vi "Eurotherm_PID_Simplified.vi"() -> ()   [LabVIEW 2013]
uses:
  <vilib>/Utility/file.llb/Write To Spreadsheet File (string).vi
  <vilib>/Utility/file.llb/Write To Spreadsheet File (DBL).vi
panel:
  in  "Ramp-Down Rate(°C/ min)":dbl
  in  "Target Setpoint (°C)":sgl format="%#.1f"
  in  "RAMP":bool
  in  "Dwell Time (min)":dbl
  in  "Ramp-Up Rate (°C/ min)":dbl
  in  "SET":bool
  in  "DELAY":u32=300 caption="ms"
  in  "Save Button":bool
  in  "File Path":path
  in  "Sample":string
  in  "User":string
  out "Time":dbl caption="(s)"
  in  "Setpoint Value":sgl min=0 max=1300 format="%.3f"
  in  "SET PID":bool
  in  "P":sgl=1.0
  in  "I":u32=10000
  in  "D":u32=1000
  in  "Controller Mode":u8(ring) items=["Auto", "Manual"]
  in  "stop":bool
  out "Temperature":cluster{dbl[], sgl[]}(graph)
  out "Temperature":sgl caption="°C" format="%.3g"
  in  "Unit":u8=1
  in  "VISA resource name":refnum<visa-resource-name>="COM4"
  # "Configuration - Requires Restart"
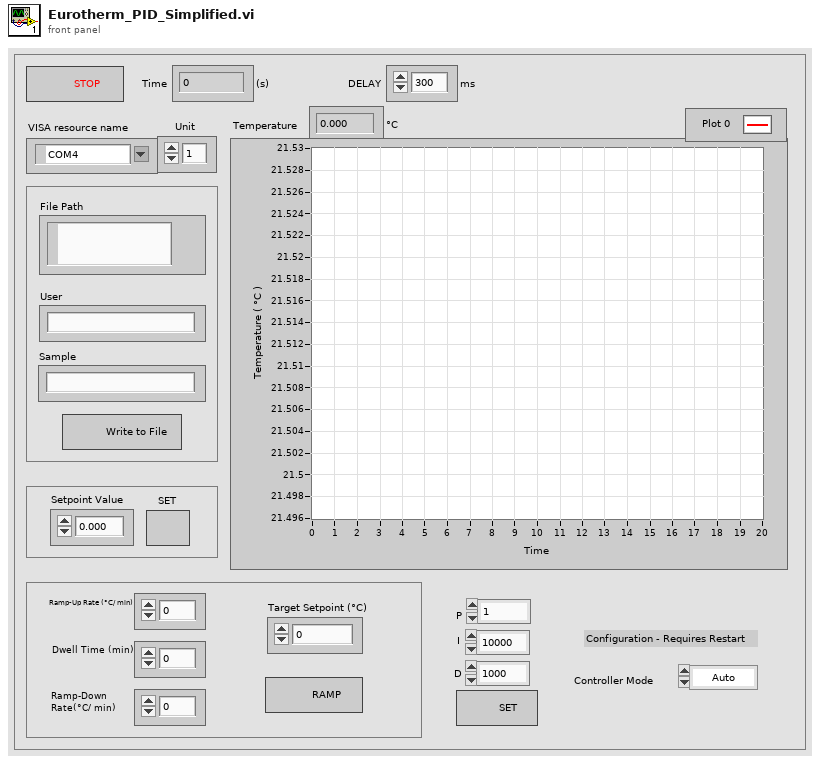
[diagram p1: front panel]
types:
  T1 = cluster{"Baud Rate (9600)":u32, "Parity (0: None)":u16, "Break Length (0)":u16}
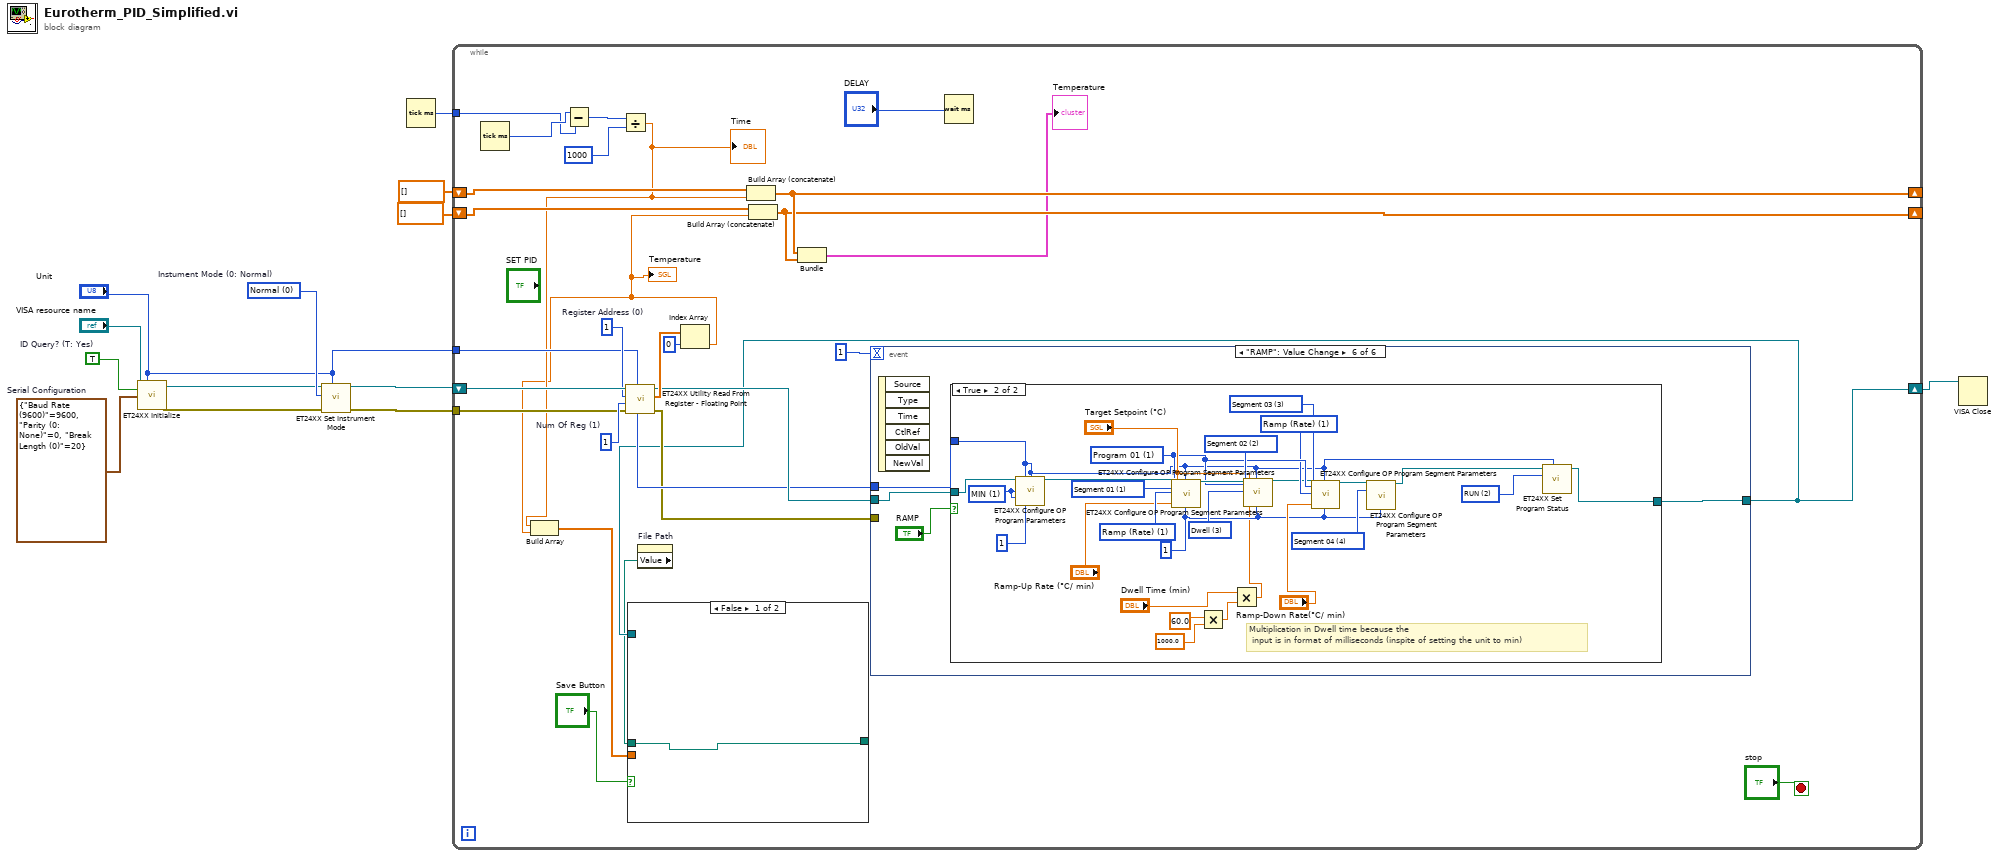
[diagram p0: block diagram]
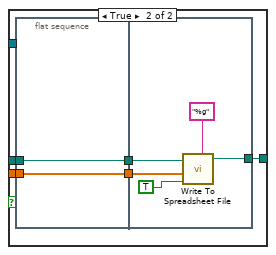
[diagram p2: hidden frame]
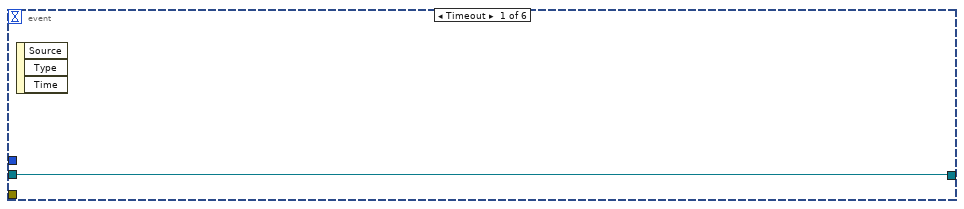
[diagram p3: hidden frame]
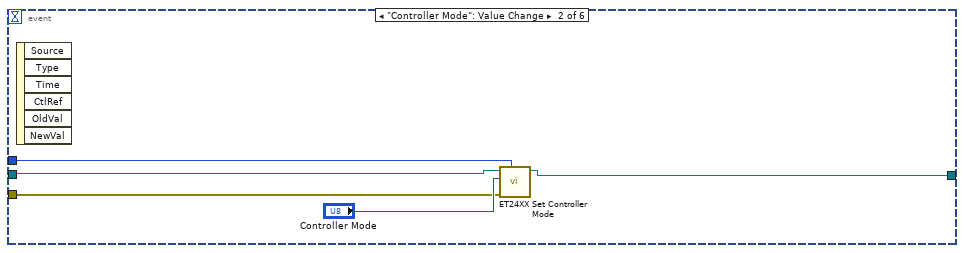
[diagram p4: hidden frame]
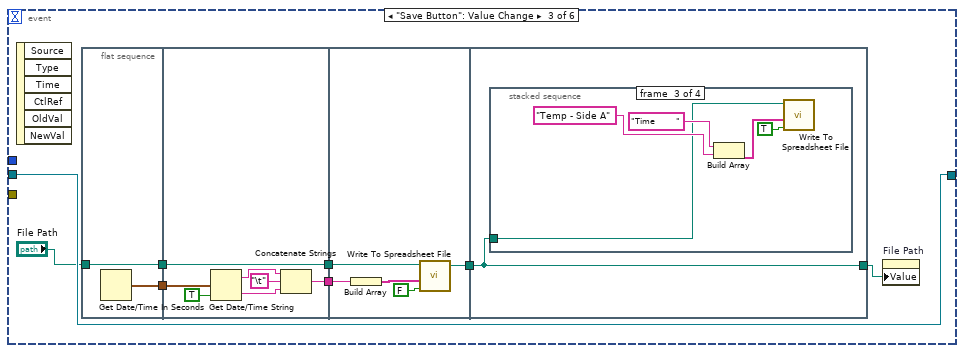
[diagram p5: hidden frame]
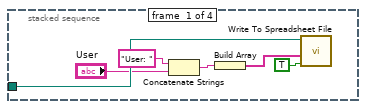
[diagram p6: hidden frame]
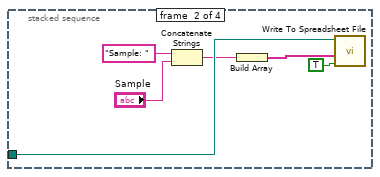
[diagram p7: hidden frame]
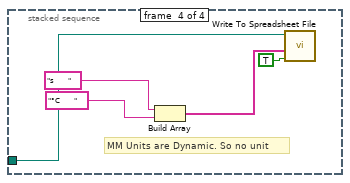
[diagram p8: hidden frame]
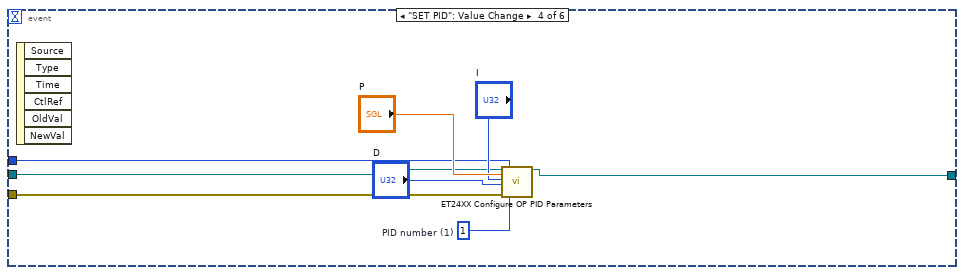
[diagram p9: hidden frame]
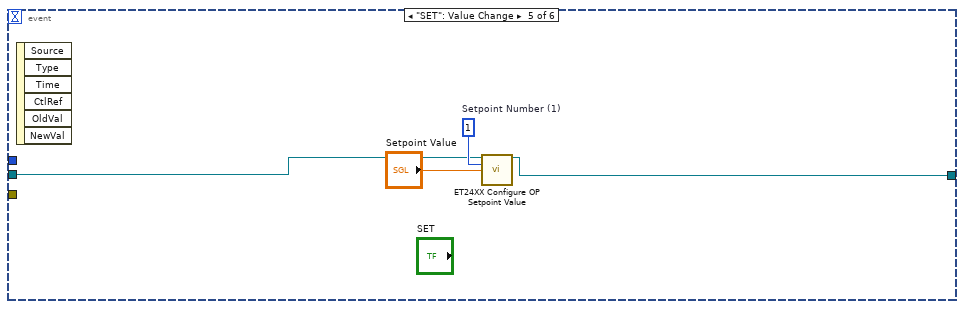
[diagram p10: hidden frame]
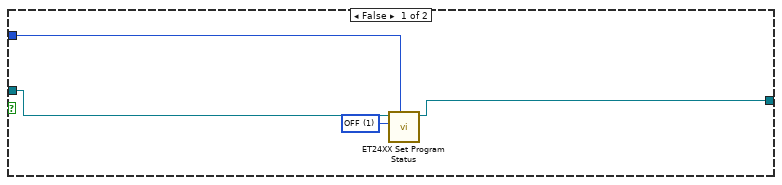
[diagram p11: hidden frame]
diagram:
  w10 = T1 {"Baud Rate (9600)"=9600, "Parity (0: None)"=0, "Break Length (0)"=20}  # Serial Configuration
  w12 = TRUE  # ID Query? (T: Yes)
  w13 = u8 0 items=["Normal", "StandBy", "Configuration"]  # Instument Mode (0: Normal)
  n1 = call <userlib>:"ET24XX Initialize.vi"("VISA resource name"="VISA resource name", "Unit Address (1)"="Unit", "ID Query? (T: Yes)"=w12, "Serial Configuration"=w10) -> ("VISA resource name out"=w2:refnum<visa-resource-name>, "error out"=w1:errorcluster)  [unwired: 10 in]
  n2 = call <userlib>:"ET24XX Set Instrument Mode.vi"("Unit Address (1)"="Unit", "error in (no error)"=w1, "Instrument Mode (0: Normal)"=w13, "VISA resource name"=w2) -> ("error out"=w3:errorcluster, "VISA resource name out"=w4:refnum<visa-resource-name>)  [unwired: 6 in]
  n3 = Tick Count (ms)() -> (millisecond timer value=w7:u32)
  n4 = while {
    tunnel: "Unit" -> [w26]
    shift-right: [w30] -> _
    shift-left: sgl[] [] -> [w35]
    tunnel: w7 -> [w17]
    shift-right: [w31] -> _
    shift-left: dbl[] [] -> [w32]
    shift-right: [w15] -> w5
    shift-left: w4 -> [w40]
    tunnel: w3 -> [w25]
    stop <- "stop" stop-if-true
    w38 = u16 1  # Num Of Reg (1)
    w39 = u16 1  # Register Address (0)
    n5 = Tick Count (ms)() -> (millisecond timer value=w18:u32)
    n6 = Subtract(x=w18, y=w17) -> (x-y=w34:u32)
    n7 = Divide(x=w34, y=u32 1000) -> (x/y=w22:dbl)
    "Time" <- w22
    n8 = call <userlib>:"ET24XX Utility Read From Register - Floating Point.vi"("Unit Address (1)"=w26, "error in (no error)"=w25, "Num Of Reg (1)"=w38, "Register Address (0)"=w39, "VISA session"=w40) -> ("error out"=w24:errorcluster, "Data"=w37:sgl[], "dup VISA session"=w27:refnum<visa-resource-name>)  [unwired: 4 in]
    n9 = property on="File Path" class="Path"() -> ("Value"=w14:path)  [unwired: 2 in, 2 out]
    n10 = Index Array(array=w37, index=0) -> (element=w21:sgl)
    "Temperature" <- w21
    n11 = Build Array(w22, w21) -> (w20:dbl[])
    n12 = Build Array (concatenate)(w32, w22) -> (w31:dbl[])
    n13 = Build Array (concatenate)(w35, w21) -> (w30:sgl[])
    n14 = Bundle(w31, w30) -> (→"Temperature":cluster{dbl[], sgl[]})  [unwired: 1 in]
    n15 = event shown="[5] \"RAMP\": Value Change" {
      selector: _ -> [_ _ _ _ _ _]
      dyn-events: _ -> [_ _ _ _ _ _]
      timeout: 1 -> [_ _ _ _ _ _]
      tunnel: w27 -> [w54 w59 w62 w108 w115 w120]
      tunnel: [w54 w57 w62 w107 w114 w118] -> w15
      tunnel: w26 -> [_ w56 _ w106 _ w119]
      tunnel: w24 -> [_ w55 _ w105 _ _]
      event Timeout {
        n16 = event-data() -> ()  [unwired: 1 in, 3 out]
      }
      event "Controller Mode": Value Change {
        n17 = event-data() -> ()  [unwired: 1 in, 6 out]
        n18 = call <userlib>:"ET24XX Set Controller Mode.vi"("Unit Address (1)"=w56, "error in (no error)"=w55, "Controller Mode (0: Auto)"="Controller Mode", "VISA resource name"=w59) -> ("VISA resource name out"=w57:refnum<visa-resource-name>)  [unwired: 6 in, 1 out]
      }
      event "Save Button": Value Change {
        n19 = event-data() -> ()  [unwired: 1 in, 6 out]
        n20 = flat-sequence {
          tunnel: [w68] -> w67
          tunnel: [w69] -> w66
          tunnel: "File Path" -> [w69]
          tunnel: w67 -> [w74]
          tunnel: [w73] -> w65
          tunnel: [w70] -> w64
          tunnel: w66 -> [w70]
          tunnel: w65 -> [w80]
          tunnel: w64 -> [w78]
          tunnel: [w77] -> w63
          tunnel: [w82] -> w60
          tunnel: w63 -> [w82]
          frame #0 {
            n21 = Get Date/Time In Seconds() -> (seconds since 1Jan1904=w68:timestamp)
          }
          frame #1 {
            n22 = Get Date/Time String(seconds (now)=w74, want seconds? (F)=TRUE) -> (date string=w76:string, time string=w72:string)  [unwired: 1 in]
            n23 = Concatenate Strings(w76, "\t", w72) -> (w73:string)
          }
          frame #2 {
            n24 = Build Array(w80) -> (w79:string[])
            n25 = call-poly <vilib>:"Write To Spreadsheet File.vi"("append to file? (new file:F)"=FALSE ("transpose? (no:F)"), "1D data"=w79, "file path (dialog if empty)"=w78) -> ("new file path (Not A Path if cancelled)"=w77:path)  [unwired: 5 in]
          }
          frame #3 {
            n26 = stacked-sequence {
              tunnel: w82 -> [w86 w92 w95 w102]
              frame #0 {
                n27 = Concatenate Strings("User: ", "User") -> (w85:string)
                n28 = Build Array(w85) -> (w87:string[])
                n29 = call-poly <vilib>:"Write To Spreadsheet File.vi"("append to file? (new file:F)"=TRUE ("transpose? (no:F)"), "1D data"=w87, "file path (dialog if empty)"=w86) -> ()  [unwired: 5 in, 1 out]
              }
              frame #1 {
                n30 = Concatenate Strings("Sample: ", "Sample") -> (w91:string)
                n31 = Build Array(w91) -> (w93:string[])
                n32 = call-poly <vilib>:"Write To Spreadsheet File.vi"("append to file? (new file:F)"=TRUE ("transpose? (no:F)"), "1D data"=w93, "file path (dialog if empty)"=w92) -> ()  [unwired: 5 in, 1 out]
              }
              frame #2 {
                n33 = Build Array("Time       ", "Temp - Side A") -> (w98:string[])
                n34 = call-poly <vilib>:"Write To Spreadsheet File.vi"("append to file? (new file:F)"=TRUE ("transpose? (no:F)"), "1D data"=w98, "file path (dialog if empty)"=w95) -> ()  [unwired: 5 in, 1 out]
              }
              frame #3 {
                # "MM Units are Dynamic. So no unit"
                n35 = Build Array("s       ", "°C       ") -> (w103:string[])
                n36 = call-poly <vilib>:"Write To Spreadsheet File.vi"("append to file? (new file:F)"=TRUE ("transpose? (no:F)"), "1D data"=w103, "file path (dialog if empty)"=w102) -> ()  [unwired: 5 in, 1 out]
              }
            }
          }
        }
        n37 = property on="File Path" class="Path"("Value"=w60) -> ()  [unwired: 2 in, 2 out]
      }
      event "SET PID": Value Change {
        w112 = i16 1  # PID number (1)
        n38 = event-data() -> ()  [unwired: 1 in, 6 out]
        n39 = call <userlib>:"ET24XX Configure OP PID Parameters.vi"("VISA resource name"=w108, "Proportional Band (1)"="P", "Integral Time (ms) (0)"="I", "Derivative Time (ms) (0)"="D", "error in (no error)"=w105, "Unit Address (1)"=w106, "PID number (1)"=w112) -> ("VISA resource name out"=w107:refnum<visa-resource-name>)  [unwired: 11 in, 1 out]
      }
      event "SET": Value Change {
        w116 = i16 1  # Setpoint Number (1)
        n40 = event-data() -> ()  [unwired: 1 in, 6 out]
        n41 = call <userlib>:"ET24XX Configure OP Setpoint Value.vi"("VISA resource name"=w115, "Setpoint Number (1)"=w116, "Setpoint Value (0)"="Setpoint Value") -> ("VISA resource name out"=w114:refnum<visa-resource-name>)  [unwired: 11 in, 1 out]
      }
      event "RAMP": Value Change {
        n42 = event-data() -> ()  [unwired: 1 in, 6 out]
        n43 = case shown="True" "RAMP" {
          tunnel: w120 -> [w124 w150]
          tunnel: w119 -> [w123 w138]
          tunnel: [w121 w151] -> w118
          frame False {
            w122 = u8 1 items=["OFF"=1, "RUN"=2, "HOLD"=4] ("Program Status (1: OFF)")
            n44 = call <userlib>:"ET24XX Set Program Status.vi"("Unit Address (1)"=w123, "Program Status (1: OFF)"=w122, "VISA resource name"=w124) -> ("VISA resource name out"=w121:refnum<visa-resource-name>)  [unwired: 7 in, 1 out]
          }
          frame True {
            w133 = u16 4 items=["Segment 01"=1, "Segment 02"=2, "Segment 03"=3, "Segment 04"=4, "Segment 05"=5, "Segment 06"=6, "Segment 07"=7, "Segment 08"=8, "Segment 09"=9, "Segment 10"=10, "Segment 11"=11, "Segment 12"=12, "Segment 13"=13, "Segment 14"=14, "Segment 15"=15, "Segment 16"=16] ("Selected Segment Number \n(1: Segment1)")
            w130 = u16 1 ("Sub-Program Cycles (0)")
            w139 = u16 3 items=["Segment 01"=1, "Segment 02"=2, "Segment 03"=3, "Segment 04"=4, "Segment 05"=5, "Segment 06"=6, "Segment 07"=7, "Segment 08"=8, "Segment 09"=9, "Segment 10"=10, "Segment 11"=11, "Segment 12"=12, "Segment 13"=13, "Segment 14"=14, "Segment 15"=15, "Segment 16"=16] ("Selected Segment Number \n(1: Segment1)")
            w140 = u8 1 items=["End", "Ramp (Rate)", "Ramp (Time to Target)", "Dwell", "Step", "Call"] ("Segment Type (0: End)")
            w143 = u8 3 items=["End", "Ramp (Rate)", "Ramp (Time to Target)", "Dwell", "Step", "Call"] ("Segment Type (0: End)")
            w144 = u16 2 items=["Segment 01"=1, "Segment 02"=2, "Segment 03"=3, "Segment 04"=4, "Segment 05"=5, "Segment 06"=6, "Segment 07"=7, "Segment 08"=8, "Segment 09"=9, "Segment 10"=10, "Segment 11"=11, "Segment 12"=12, "Segment 13"=13, "Segment 14"=14, "Segment 15"=15, "Segment 16"=16] ("Selected Segment Number \n(1: Segment1)")
            w146 = u8 1 items=["End", "Ramp (Rate)", "Ramp (Time to Target)", "Dwell", "Step", "Call"] ("Segment Type (0: End)")
            w141 = u16 1 items=["Program 01"=1, "Program 02"=2, "Program 03"=3, "Program 04"=4, "Program 05"=5, "Program 06"=6, "Program 07"=7, "Program 08"=8, "Program 09"=9, "Program 10"=10, "Program 11"=11, "Program 12"=12, "Program 13"=13, "Program 14"=14, "Program 15"=15, "Program 16"=16, "Program 17"=17, "Program 18"=18, "Program 19"=19, "Program 20"=20] ("Selected Program Number \n(1: Program 01)")
            w147 = u16 1 items=["Segment 01"=1, "Segment 02"=2, "Segment 03"=3, "Segment 04"=4, "Segment 05"=5, "Segment 06"=6, "Segment 07"=7, "Segment 08"=8, "Segment 09"=9, "Segment 10"=10, "Segment 11"=11, "Segment 12"=12, "Segment 13"=13, "Segment 14"=14, "Segment 15"=15, "Segment 16"=16] ("Selected Segment Number \n(1: Segment1)")
            w149 = u8 1 items=["SEC", "MIN", "HOUR"] ("Ramp Time Units (0: SEC)")
            w152 = u8 2 items=["OFF"=1, "RUN"=2, "HOLD"=4] ("Program Status (1: OFF)")
            # "Multiplication in Dwell time because the\n input is in format of milliseconds (inspite of setting the unit to min)"
            n45 = call <userlib>:"ET24XX Configure OP Program Parameters.vi"("VISA resource name"=w150, "Unit Address (1)"=w138, "Program number (1)"=w138, "Ramp Time Units (0: SEC)"=w149, "Dwell Time Units (0: SEC)"=w149, "Program Cycles (0)"=u16 1) -> ("VISA resource name out"=w148:refnum<visa-resource-name>)  [unwired: 8 in, 1 out]
            n46 = call "ET24XX Configure OP Program Segment Parameters.vi"("VISA resource name"=w148, "Selected Program Number \n(1: Program 01)"=w141, "Selected Segment Number \n(1: Segment1)"=w147, "Segment Type (0: End)"=w146, "Ramp Rate (1)"="Ramp-Up Rate (°C/ min)", "Target Setpoint (0)"="Target Setpoint (°C)", "Unit Address (1)"=w138, "Sub-Program Cycles (0)"=w130) -> ("VISA resource name out"=w145:refnum<visa-resource-name>)  [unwired: 18 in, 1 out]
            n47 = Multiply(x=60.0, y=1000.0) -> (x*y=w126:dbl)
            n48 = Multiply(x="Dwell Time (min)", y=w126) -> (x*y=w125:dbl)
            n49 = call "ET24XX Configure OP Program Segment Parameters.vi"("VISA resource name"=w145, "Selected Program Number \n(1: Program 01)"=w141, "Selected Segment Number \n(1: Segment1)"=w144, "Segment Type (0: End)"=w143, "Target Setpoint (0)"="Target Setpoint (°C)", "Duration (N/A)"=w125, "Unit Address (1)"=w138, "Sub-Program Cycles (0)"=w130) -> ("VISA resource name out"=w137:refnum<visa-resource-name>)  [unwired: 18 in, 1 out]
            n50 = call "ET24XX Configure OP Program Segment Parameters.vi"("VISA resource name"=w137, "Selected Program Number \n(1: Program 01)"=w141, "Selected Segment Number \n(1: Segment1)"=w139, "Segment Type (0: End)"=w140, "Ramp Rate (1)"="Ramp-Down Rate(°C/ min)", "Unit Address (1)"=w138, "Sub-Program Cycles (0)"=w130) -> ("VISA resource name out"=w135:refnum<visa-resource-name>)  [unwired: 19 in, 1 out]
            n51 = call "ET24XX Configure OP Program Segment Parameters.vi"("VISA resource name"=w135, "Selected Segment Number \n(1: Segment1)"=w133, "Sub-Program Cycles (0)"=w130) -> ("VISA resource name out"=w134:refnum<visa-resource-name>)  [unwired: 23 in, 1 out]
            n52 = call <userlib>:"ET24XX Set Program Status.vi"("Unit Address (1)"=w138, "Program Status (1: OFF)"=w152, "VISA resource name"=w134) -> ("VISA resource name out"=w151:refnum<visa-resource-name>)  [unwired: 7 in, 1 out]
          }
        }
      }
    }
    n53 = case shown="False" "Save Button" {
      tunnel: [w41 w46] -> _
      tunnel: w14 -> [w41 w44]
      tunnel: w20 -> [_ w42]
      tunnel: w15 -> [_ _]
      frame False {
      }
      frame True {
        n54 = flat-sequence {
          tunnel: [w48] -> w45
          tunnel: w44 -> [w48]
          tunnel: [w47] -> w43
          tunnel: w42 -> [w47]
          tunnel: [w52] -> w46
          tunnel: w45 -> [w51]
          tunnel: w43 -> [w50]
          frame #0 {
          }
          frame #1 {
            n55 = call-poly <vilib>:"Write To Spreadsheet File.vi"("format (%.3f)"="%g", "append to file? (new file:F)"=TRUE ("transpose? (no:F)"), "1D data"=w50, "file path (dialog if empty)"=w51) -> ("new file path (Not A Path if cancelled)"=w52:path)  [unwired: 4 in]
          }
        }
      }
    }
    n56 = Wait (ms)(milliseconds to wait="DELAY") -> ()  [unwired: 1 out]
  }
  n57 = VISA Close(VISA resource name=w5) -> ()  [unwired: 1 in, 1 out]
